vi "4_2.vi"() -> ()   [LabVIEW 2015]
panel:
  out "[0] 6":u8
  out "[0] 5":u8
  out "[0] 4":u8
  out "[0] 3":u8
  out "[0] 2":u8
  out "[0]":u8
  # "7"
  # "13"
  # "26"
  # "37"
  # "47"
  # "42"
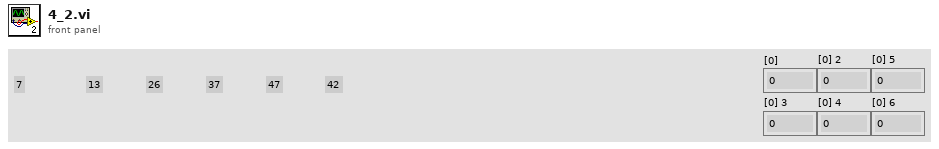
[diagram p1: front panel]
types:
  T1 = cluster{"[0]":u8, "[1]":u8, "[2]":u8, "[3]":u8, "[4]":u8, "[5]":u8, "[6]":u8, "[7]":u8, "[8]":u8}
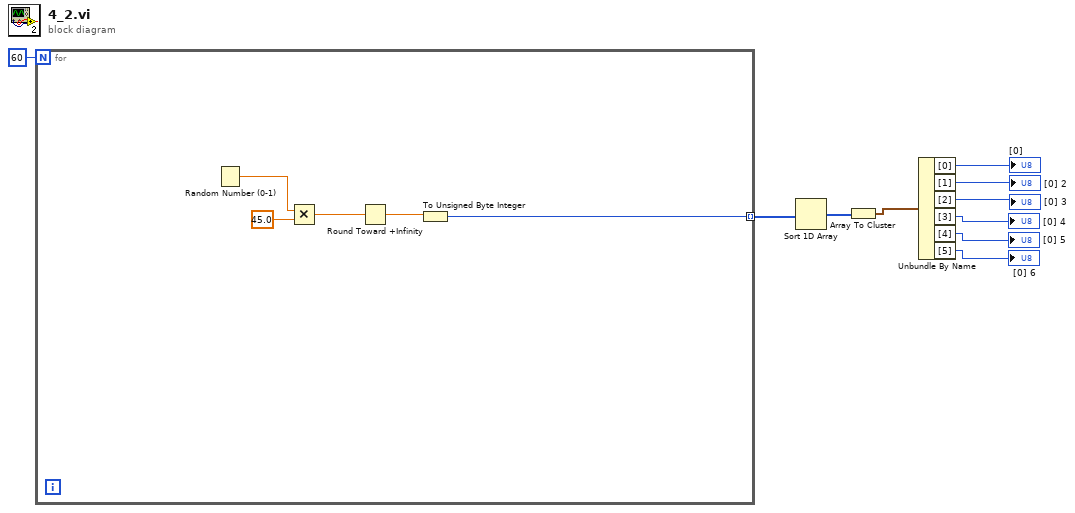
[diagram p0: block diagram]
diagram:
  n1 = for {
    N: 60 -> [_]
    tunnel: [w11] -> w9 mode=indexing
    n2 = Random Number (0-1)() -> (number: 0 to 1=w15:dbl)
    n3 = Multiply(x=w15, y=45.0) -> (x*y=w13:dbl)
    n4 = Round Toward +Infinity(x=w13) -> (ceil(x): smallest int >= x=w12:dbl)
    n5 = To Unsigned Byte Integer(number=w12) -> (unsigned 8bit integer=w11:u8)
  }
  n6 = Sort 1D Array(array=w9) -> (sorted array=w8:u8[])
  n7 = Array To Cluster(array=w8) -> (cluster=w7:T1)
  n8 = Unbundle By Name(w7) -> ("[0]"=→"[0]":u8, "[1]"=→"[0] 2":u8, "[2]"=→"[0] 3":u8, "[3]"=→"[0] 4":u8, "[4]"=→"[0] 5":u8, "[5]"=→"[0] 6":u8)
